vi "varToRobcomm.vi"(1 "var name":string, 2 "var value":dbl=9.5, 3 "VISA resource name":refnum<visa-resource-name>) -> (0 "VISA resource name out":refnum<visa-resource-name>)   [LabVIEW 2012]
panel:
  out "error out":errorcluster
  out "return count":u32
  out "write output":string
  out "concatenated string":string
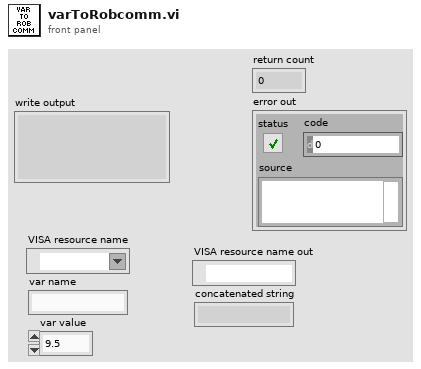
[diagram p1: front panel]
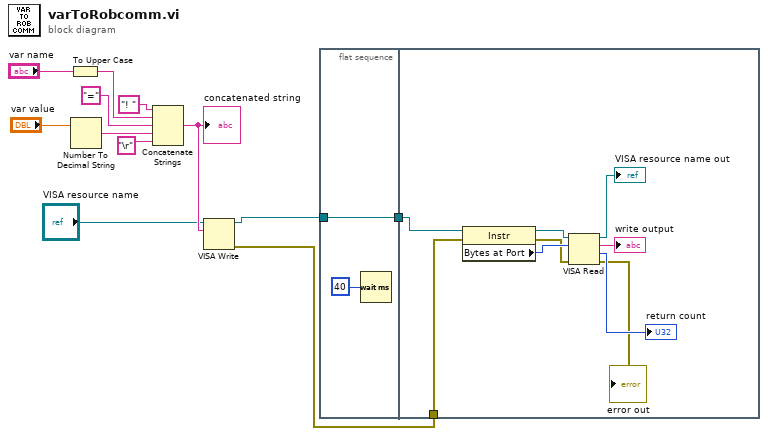
[diagram p0: block diagram]
diagram:
  n1 = To Upper Case(1:"var name") -> (0:w6:string)
  n2 = Number To Decimal String(number="var value") -> (decimal integer string=w10:string)  [unwired: 1 in]
  n3 = Concatenate Strings("! " ("write buffer"), w6, "=" ("write buffer"), w10, "\r" ("string")) -> (w12:string)
  "concatenated string" <- w12
  n4 = VISA Write(VISA resource name="VISA resource name", write buffer=w12) -> (VISA resource name out=w4:refnum<visa-resource-name>, error out=w2:errorcluster)  [unwired: 1 in, 1 out]
  n5 = flat-sequence {
    tunnel: w4 -> [w14]
    tunnel: [w14] -> w3
    tunnel: w3 -> [w21]
    tunnel: w2 -> [w17]
    frame #0 {
      n6 = Wait (ms)(milliseconds to wait=u32 40) -> ()  [unwired: 1 out]
    }
    frame #1 {
      n7 = property class="Instr"(reference=w21, error in=w17) -> (reference out=w20:refnum<visa-resource-name>, error out=w16:errorcluster, "Bytes at Port"=w19:u32)
      n8 = VISA Read(VISA resource name=w20, byte count=w19, error in (no error)=w16) -> (VISA resource name out=→"VISA resource name out":refnum<visa-resource-name>, read buffer=→"write output":string, return count=→"return count":u32, error out=→"error out":errorcluster)
    }
  }
